vi "Get owning Library.vi"(8 "Error In":errorcluster, 11 "VI Refnum":refnum<vi>) -> (0 "Error Out":errorcluster, 3 "Owning Library":refnum<vi>)   [LabVIEW 2011, in "Generator.lvlib"]
doc: "This VI returns a reference to the owning Library of <B>VI Refnum</B>."
uses:
  Generator.lvlib
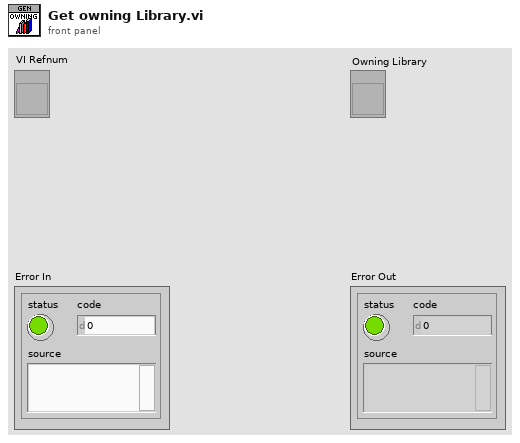
[diagram p1: front panel]
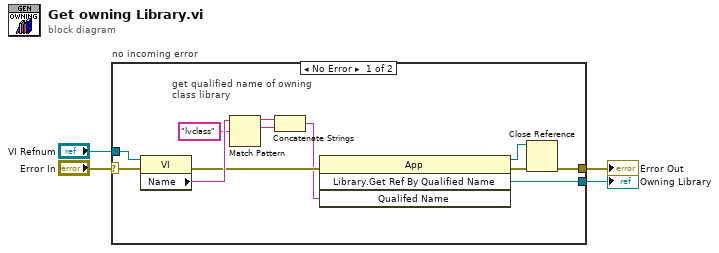
[diagram p0: block diagram]
diagram:
  n1 = case "no incoming error" shown="No Error" "Error In" {
    selector: "Error In" -> [w16 w17]
    tunnel: [w5 w17] -> w3
    tunnel: "VI Refnum" -> [w15 _]
    tunnel: [w6 _] -> w1
    frame No Error {
      # "get qualified name of owning\nclass library"
      n2 = property class="VI"(reference=w15, error in=w16) -> (error out=w10:errorcluster, "Name"=w14:string)  [unwired: 1 out]
      n3 = Match Pattern(string=w14, regular expression="lvclass") -> (before substring=w12:string, match substring=w11:string)  [unwired: 1 in, 2 out]
      n4 = Concatenate Strings(w12, w11) -> (w9:string)
      n5 = invoke class="App" method="Library.Get Ref By Qualified Name"(error in=w10, "Qualifed Name"=w9) -> (reference out=w7:refnum<vi>, error out=w8:errorcluster, "Library.Get Ref By Qualified Name"=w6:refnum<vi>)  [unwired: 2 in, 1 out]
      n6 = Close Reference(reference=w7, error in (no error)=w8) -> (error out=w5:errorcluster)
    }
    frame Error {
    }
  }
  "Error Out" <- w3
  "Owning Library" <- w1
